vi "Create TDMS File.vi"(7 "Time Stamp":timestamp, 8 "error in (no error)":errorcluster, 11 "Log file path":path) -> (0 "error out":errorcluster, 3 "TDMS ref out":refnum<k34>)   [LabVIEW 2021, in "XNET-CAN-Signal-Logger.lvlib"]
uses:
  XNET-CAN-Signal-Logger.lvlib
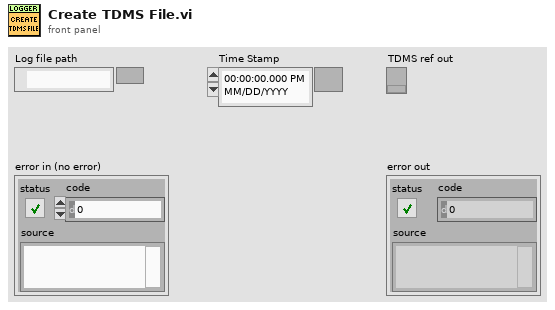
[diagram p1: front panel]
types:
  T1 = enum16{"open", "open or create", "create or replace", "create", "open (read-only)"}
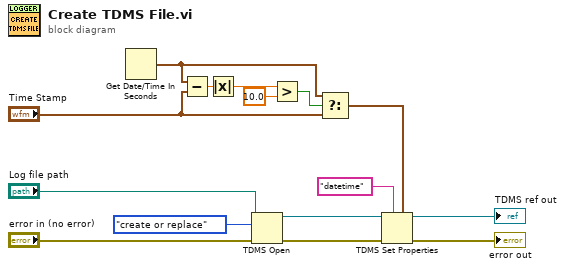
[diagram p0: block diagram]
diagram:
  n1 = Get Date/Time In Seconds() -> (seconds since 1Jan1904=w3:timestamp)
  n2 = Subtract(x=w3, y="Time Stamp") -> (x-y=w7:dbl)
  n3 = Absolute Value(x=w7) -> (abs(x)=w6:dbl)
  n4 = TDMS Open(8:"error in (no error)", 10:T1."create or replace" ("operation (0:open)"), 11:"Log file path") -> (3:w10:refnum<k34>)  [unwired: 4 in, 1 out]
  n5 = Greater?(x=w6, y=10.0) -> (0:w4:bool)
  n6 = Select(t=w3, s=w4, f="Time Stamp") -> (s? t:f=w1:timestamp)
  n7 = TDMS Set Properties(5:w1, 7:"datetime" ("property names"), 8:"error in (no error)", 11:w10) -> (0:→"error out":errorcluster, 3:→"TDMS ref out":refnum<k34>)  [unwired: 2 in, 2 out]
